vi "gun_rt_slow_upstream_datastore.vi"(10 "data_store_mode":enum16{"Set", "Get"}(ring), 11 "gun_rt_slow_upstream_data":T1={"turret"={"turret_analog"=0.0, "turret_angle"=0.0, "turret_motor"=0.0, "turret_idg_state"=enum."fault_high"}, "hood"={"hood_analog"=0.0, "hood_angle"=0.0, "hood_motor"=0.0, "hood_idg_state"=enum."fault_high"}}) -> (3 "gun_rt_slow_upstream_data out":T1={"turret"={"turret_analog"=0.0, "turret_angle"=0.0, "turret_motor"=0.0, "turret_idg_state"=enum."fault_high"}, "hood"={"hood_analog"=0.0, "hood_angle"=0.0, "hood_motor"=0.0, "hood_idg_state"=enum."fault_high"}})   [LabVIEW 2011]
uses:
  gun_rt_slow_upstream_data.ctl
  idg_trust_t.ctl
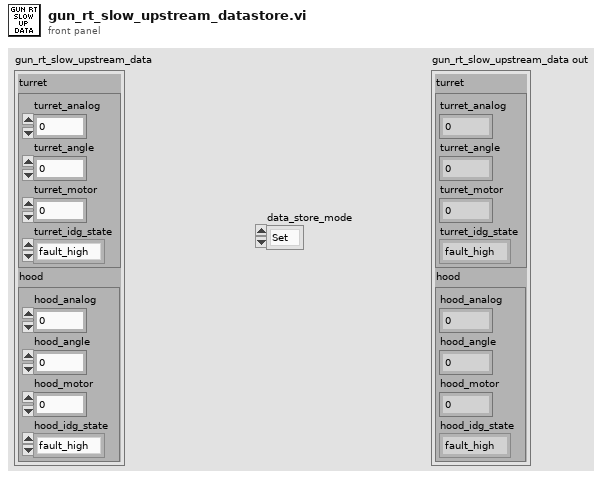
[diagram p1: front panel]
types:
  T1 = typedef "gun_rt_slow_upstream_data.ctl" = cluster{"turret":cluster{"turret_analog":dbl, "turret_angle":dbl, "turret_motor":dbl, "turret_idg_state":T2}, "hood":cluster{"hood_analog":dbl, "hood_angle":dbl, "hood_motor":dbl, "hood_idg_state":T2}}
  T2 = typedef "idg_trust_t.ctl" = enum16{"fault_move", "fault_high", "fault_low", "out_high", "out_low", "trust"}
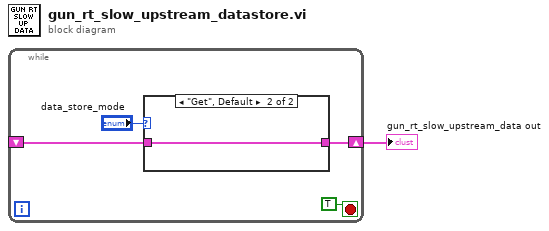
[diagram p0: block diagram]
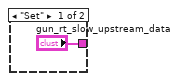
[diagram p2: hidden frame]
diagram:
  n1 = while {
    shift-right: [w3] -> w1
    shift-left: _ -> [w2]
    stop <- TRUE stop-if-true
    n2 = case shown="\"Get\", Default" "data_store_mode" {
      tunnel: ["gun_rt_slow_upstream_data" w7] -> w3
      tunnel: w2 -> [_ w7]
      frame "Set" {
      }
      frame "Get", Default {
      }
    }
  }
  "gun_rt_slow_upstream_data out" <- w1
